vi "data_ID_impact.vi"(6 "Sensor Lookup Indices":i32[](array[numeric]), 7 "Start Z_Threshold":dbl format="%#_13g", 8 "error in (no error)":errorcluster, 9 "Pkt Size":i32, 10 "Gains":dbl[](array[numeric]), 11 "Byte Stream File in":refnum<file>) -> (0 "error out":errorcluster, 2 "Sensor_Tare":dbl[][](array[numeric]), 3 "Byte Stream File out":refnum<file>, 4 "N_end":i32, 5 "N_start":i32)   [LabVIEW 2018]
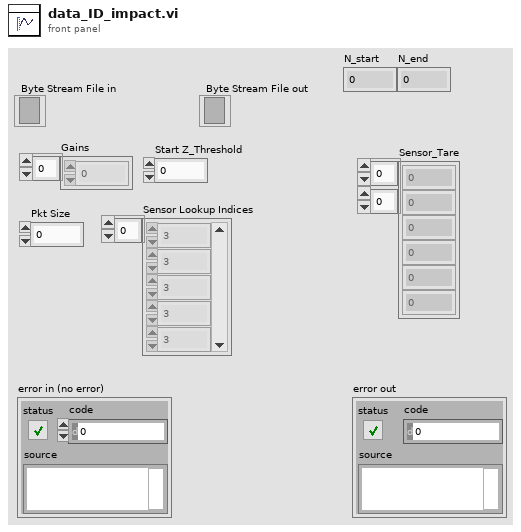
[diagram p1: front panel]
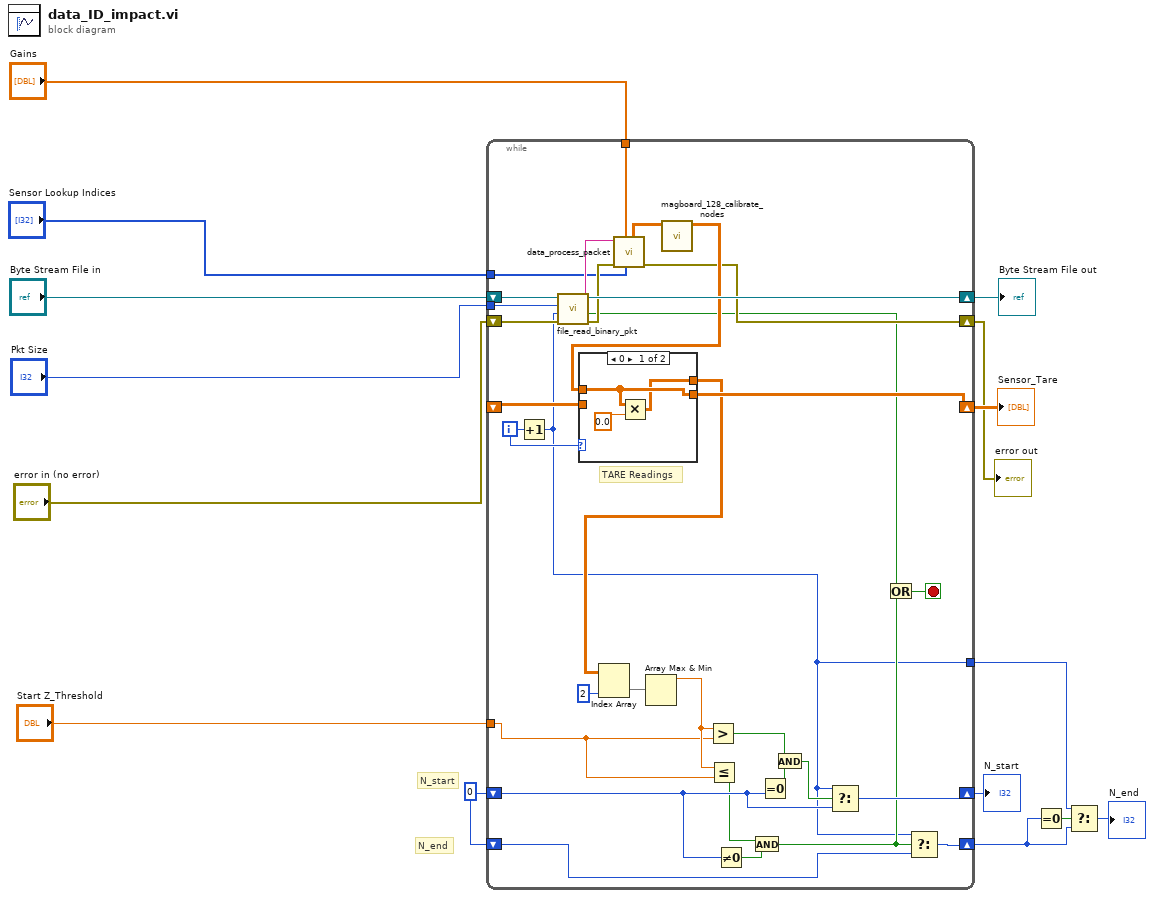
[diagram p0: block diagram]
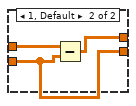
[diagram p2: hidden frame]
diagram:
  w8 = 0
  # "N_end"
  # "N_start"
  n1 = while {
    tunnel: "Pkt Size" -> [w46]
    shift-right: [w44] -> w11
    shift-left: "Byte Stream File in" -> [w47]
    shift-right: [w36] -> w13
    shift-left: "error in (no error)" -> [w43]
    shift-right: [w37] -> w15
    shift-left: _ -> [w38]
    tunnel: "Gains" -> [w35]
    shift-right: [w27] -> w7
    shift-left: w8 -> [w26]
    shift-right: [w23] -> w2
    shift-left: w8 -> [w22]
    tunnel: "Sensor Lookup Indices" -> [w18]
    tunnel: "Start Z_Threshold" -> [w17]
    tunnel: [w16] -> w3
    i -> [w45]
    stop <- w21 stop-if-true
    # "TARE Readings"
    n2 = Increment(x=w45) -> (x+1=w16:i32)
    n3 = call "file_read_binary_pkt.vi"("error in (no error)"=w43, "Packet No."=w16, "Pkt Size(bytes)"=w46, "Byte Stream File in"=w47) -> ("error out"=w41:errorcluster, "EOF?"=w20:bool, "Packet"=w42:string, "Byte Stream File out"=w44:refnum<file>)  [unwired: 4 in]
    n4 = call "data_process_packet.vi"("Sensor Lookup Indices"=w18, "Gains"=w35, "error in (no error)"=w41, "Binary Input Data"=w42) -> ("error out"=w36:errorcluster, "Sensors (uT)"=w40:dbl[][])  [unwired: 3 in, 3 out]
    n5 = call "magboard_128_calibrate_nodes.vi"("Sensor Input (mT)"=w40) -> ("Sensor Output - Position (mm)"=w39:dbl[][])  [unwired: 10 in]
    n6 = case shown="0" w45 {
      tunnel: w39 -> [w50 w53]
      tunnel: w38 -> [_ w52]
      tunnel: [w50 w52] -> w37
      tunnel: [w49 w51] -> w32
      frame 0 {
        n7 = Multiply(x=w50, y=0.0) -> (x*y=w49:dbl[][])
      }
      frame 1, Default {
        n8 = Subtract(x=w53, y=w52) -> (x-y=w51:dbl[][])
      }
    }
    n9 = Index Array(array=w32, index (col)=2 ("disabled index (col)")) -> (element=w34:dbl[])  [unwired: 1 in]
    n10 = Array Max & Min(array=w34) -> (max value=w31:dbl)  [unwired: 3 out]
    n11 = Greater?(x=w31, y=w17) -> (0:w30:bool)
    n12 = Less Or Equal?(x=w31, y=w17) -> (x <= y?=w24:bool)
    n13 = Not Equal To 0?(x=w26) -> (x != 0?=w25:bool)
    n14 = And(x=w24, y=w25) -> (x .and. y?=w19:bool)
    n15 = Equal To 0?(x=w26) -> (x = 0?=w29:bool)
    n16 = And(x=w30, y=w29) -> (x .and. y?=w28:bool)
    n17 = Select(t=w16, s=w28, f=w26) -> (s? t:f=w27:i32)
    n18 = Or(x=w20, y=w19) -> (x .or. y?=w21:bool)
    n19 = Select(t=w16, s=w19, f=w22) -> (s? t:f=w23:i32)
  }
  "Sensor_Tare" <- w15
  "error out" <- w13
  "Byte Stream File out" <- w11
  "N_start" <- w7
  n20 = Equal To 0?(x=w2) -> (x = 0?=w4:bool)
  n21 = Select(t=w3, s=w4, f=w2) -> (s? t:f=→"N_end":i32)
